vi "Stimulus Channel (G3)-Serialize.vi"(8 "error in":errorcluster, 11 "variant":variant) -> (0 "error out":errorcluster, 1 "Cluster Data Types":variant[](array[variant]), 3 "Cluster Variants":variant[](array[variant]))   [LabVIEW 2020, in "Stimulus Channel (G3).xctl"]
uses:
  Stimulus Channel (G3).xctl
  Waveform VIs/Complex Tone VIs/CT.Properties.ctl
  Waveform VIs/Complex Tone VIs/CT-Phase Enum.ctl
  Level (G3)/Level.Properties.ctl
  Level (G3)/Level Units (G3).ctl
  Full Stimulus Channel Data.ctl
  Waveform XControls/Waveform (G3)/Waveform Data.ctl
  Waveform VIs/Waveform Enum (V3).ctl
  Waveform XControls/Tone (G3)/Tone.Properties.ctl
  Waveform VIs/Pulse Train VIs/Pulse Train Params.ctl
  Waveform VIs/Pulse Train VIs/Pulse Polarity.ctl
  Waveform VIs/Pulse Train VIs/PT-Continuous State.ctl
  Waveform VIs/Noise VIs/Noise (G3).ctl
  Waveform VIs/Noise VIs/Noise (G3).Properties.ctl
  Waveform VIs/Noise VIs/Noise (G3).Data.ctl
  Waveform VIs/File VIs/StimFile-Params.ctl
  Waveform VIs/FM Sweep VIs/FM Sweep Params.ctl
  Waveform VIs/Chirp Train VIs/Chirp Train.ctl
  Waveform VIs/Chirp Train VIs/Chirp Train Params.ctl
  Waveform VIs/Complex Tone VIs/CT-Params.ctl
  Waveform VIs/Complex Tone VIs/CT-Runtime Data.ctl
  Waveform XControls/FM Tone/Data.ctl
  Waveform XControls/Vowel/Vowel.Properties.ctl
  Waveform VIs/Ramp VIs/Ramp.Properties.ctl
  Filter (G3)/Filter Data.ctl
  Filter (G3)/Filter Type.ctl
  Filter VIs/Filter-Bandwidth Units.ctl
  Controls/Burst XCtl/Burst Data.ctl
  Level (G3)/Level Data.ctl
  Advanced Options (G3)/Advanced Options (G3).ctl
  Modulation VIs/SAM VIs/SAM Params.ctl
  Typedefs/Destination.ctl
  Modulation VIs/SAM VIs/SAM.Properties.ctl
  Controls/Waveform XCtl/Waveform Enum.ctl
  Waveform VIs/Tone VIs/Tone.Properties.ctl
  Waveform VIs/Pulse Train VIs/Pulse Train.Properties.ctl
  Waveform VIs/File VIs/File.Properties.ctl
  Waveform VIs/FM Sweep VIs/FMSweep.Properties.ctl
  Waveform VIs/Chirp Train VIs/Chirp Train.Properties.ctl
  Waveform XControls/FM Tone/FM.Properties.ctl
  Waveform XControls/Waveform (G3)/Waveform (G3).xctl
  Filter (G3)/Filter (G3).xctl
  Controls/Burst XCtl/Burst Control.xctl
  Level (G3)/Level (G3).xctl
  <vilib>/Utility/Data Type/NI_Data Type.lvlib
  Advanced Options (G3)/Advanced Options (G3).xctl
  Waveform XControls/Tone (G3)/Tone (G3).xctl
  Waveform XControls/FM Tone/FM Tone.xctl
  Waveform XControls/Vowel/Vowel.xctl
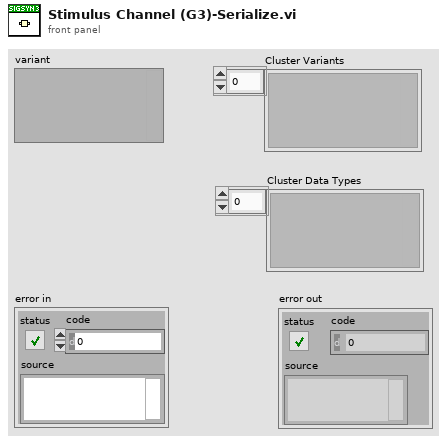
[diagram p1: front panel]
types:
  T1 = typedef "CT.Properties.ctl" = cluster{"F0 (Hz)":dbl, "Band":cluster{"Flow (Hz)":dbl, "Fhigh (Hz)":dbl}, "Phase":T2, "Min F0 (Hz)":dbl, "Max F0 (Hz)":dbl, "ContinRandPhase":bool, "Max peak factor":dbl, "Max mod depth":dbl, "MinHarmNum":i32, "MaxHarmNum":i32, "Level Mode":enum16{"per component", "overall rms"}}
  T2 = typedef "CT-Phase Enum.ctl" = enum16{"Cosine", "Random", "Alternating"}
  T3 = typedef "Level.Properties.ctl" = cluster{"Level":dbl, "Units":T4}
  T4 = typedef "Level (G3).xctl/Level Units (G3).ctl" = enum16{"dB atten", "dB SPL", "dB re 1 Vrms", "dB V/Hz½", "mW", "dB HL", "Volts", "dB mW"}
  T5 = typedef "Stimulus Channel (G3).xctl/Full Stimulus Channel Data.ctl" = cluster{"Waveform":T6, "Filter":T24, "Burst":T27, "Level":T28, "Name":string, "Advanced":T29, "SAM":T30, "Destination":T31}
  T6 = typedef "Waveform (G3).xctl/Waveform Data.ctl" = cluster{"Type":T7, "Tone":T8, "Pulse Train":T9, "Noise":T12, "File":T15, "FMSweep":T16, "Chirp Train":T17, "Complex Tone":cluster{"Params":T19, "Data":T20}, "FM":T21, "Vowel":T22, "Ramp":T23}
  T7 = typedef "Waveform Enum (V3).ctl" = enum16{"OFF", "Tone", "Noise", "Pulse Train", "File", "FM Sweep", "Chirp Train", "Complex Tone", "FM Tone", "Vowel", "Ramp"}
  T8 = typedef "Tone (G3).xctl/Tone.Properties.ctl" = cluster{"Frequency (kHz)":dbl, "Phase (cycles)":dbl, "Random phase":bool}
  T9 = typedef "Pulse Train Params.ctl" = cluster{"Pulse width (us)":dbl, "Pulse rate (Hz)":dbl, "Gap (ms)":dbl, "Polarity":T10, "PT State":T11, "Asynch":bool}
  T10 = typedef "Pulse Polarity.ctl" = enum16{"POS", "NEG", "POS-NEG", "NEG-POS"}
  T11 = typedef "PT-Continuous State.ctl" = cluster{"Template":dbl[], "Nperiod":i32, "Index":i32, "Pulse Rate (Hz)":dbl, "Phase (cycles)":dbl, "Noff":i32}
  T12 = typedef "Noise (G3).ctl" = cluster{"Properties":T13, "Data":T14}
  T13 = typedef "Noise (G3).Properties.ctl" = cluster{"InvFilt":bool, "Aweight":bool, "Seed":i32, "Tokens":i32, "Brickwall":bool}
  T14 = typedef "Noise (G3).Data.ctl" = cluster{"TokenNum":i32}
  T15 = typedef "StimFile-Params.ctl" = cluster{"Filename":path, "Signal":dbl[], "Channel":i32, "stream":bool, "offset":i32, "nreps":i32, "loops":i32, "Randomize":bool, "order":i32[], "Seed":i32, "Tokens":i32}
  T16 = typedef "FM Sweep Params.ctl" = cluster{"Rate (oct/s)":dbl, "Fmin (Hz)":dbl, "Fmax (Hz)":dbl, "Ramp (ms)":dbl, "Linear":bool}
  T17 = typedef "Chirp Train.ctl" = cluster{"Params":T18, "Data":cluster{"WF":dbl[]}}
  T18 = typedef "Chirp Train Params.ctl" = cluster{"Fmin (kHz)":dbl, "Fmax (kHz)":dbl, "Compensate":bool, "Duration (ms)":dbl}
  T19 = typedef "CT-Params.ctl" = cluster{"F0 (Hz)":dbl, "Band":cluster{"Flow (Hz)":dbl, "Fhigh (Hz)":dbl}, "Phase":T2, "Min F0 (Hz)":dbl, "Max F0 (Hz)":dbl, "ContinRandPhase":bool, "Max peak factor":dbl, "Max mod depth":dbl, "MinHarmNum":i32, "MaxHarmNum":i32, "Level Mode":enum16{"per component", "overall rms"}, "% jitter":dbl}
  T20 = typedef "CT-Runtime Data.ctl" = cluster{"Ncomp":i32, "MinHarm":i32, "Phase":dbl[], "Amplitude":dbl[], "Npts/frame":i32, "Last F0":dbl, "Fmin":dbl, "Fmax":dbl, "Lslope":dbl, "randphase":bool, "overall rms":bool, "fmult":dbl[], "jittered":bool}
  T21 = typedef "FM Tone.xctl/Data.ctl" = cluster{"Carrier (kHz)":dbl, "ModRate (Hz)":dbl, "Depth (Hz)":dbl, "Phase (cycles)":dbl}
  T22 = typedef "Vowel.xctl/Vowel.Properties.ctl" = cluster{"Freqs":string, "Set level":enum16{"Total", "Per component"}, "Freq":dbl[], "weights":dbl[]}
  T23 = typedef "Ramp.Properties.ctl" = cluster{"Duration (ms)":dbl}
  T24 = typedef "Filter (G3).xctl/Filter Data.ctl" = cluster{"Type":T25, "CF (kHz)":dbl, "BW (kHz)":dbl, "Cascade":bool, "Quadrature":bool, "Scale Factor":dbl, "Stages":cluster{"IIR Filter":cluster{"filter structure":enum32{"IIR 2nd Order", "IIR 4th Order"}, "Reverse Coefficients":dbl[], "Forward Coefficients":dbl[]}, "State":dbl[]}[], "Class":enum16{"Elliptic", "Butterworth"}, "Order":i32, "BWUnits":T26}
  T25 = typedef "Filter (G3).xctl/Filter Type.ctl" = enum16{"OFF", "Lowpass", "Highpass", "Bandpass", "Bandstop"}
  T26 = typedef "Filter-Bandwidth Units.ctl" = enum16{"Linear", "Octaves", "Min-Max"}
  T27 = typedef "Burst Control.xctl/Burst Data.ctl" = cluster{"Active":bool, "Delay (ms)":dbl, "Duration (ms)":dbl, "Ramp (ms)":dbl, "Rate (Hz)":dbl, "Trepeat (ms)":dbl, "Repeat":bool}
  T28 = typedef "Level (G3).xctl/Level Data.ctl" = cluster{"Level":dbl, "Units":T4, "Max":dbl, "Data":cluster{"Multiplier":dbl, "Cal File":path, "Cal":cluster{"Freq (Hz)":dbl[], "Mag (dB SPL)":dbl[], "Phase (deg)":dbl[]}, "audiogram":path}}
  T29 = typedef "Advanced Options (G3).xctl/Advanced Options (G3).ctl" = cluster{"AltPol":bool, "Var":string, "Expr":string}
  T30 = typedef "SAM Params.ctl" = cluster{"Active":bool, "Frequency (Hz)":dbl, "Depth":dbl, "Init Phase (cycles)":dbl, "phase (degrees)":dbl, "Asynch":bool}
  T31 = typedef "Destination.ctl" = cluster{"Name":string, "Num":i32}
  T32 = typedef "Waveform Enum.ctl" = enum16{"OFF", "Tone", "Noise", "Pulse Train", "File", "FM Sweep", "Chirp Train", "Complex Tone", "FM Tone", "Moving Ripple"}
  T33 = typedef "Tone.Properties.ctl" = cluster{"Frequency (kHz)":dbl, "Phase (cycles)":dbl, "Random phase":bool}
  T34 = typedef "Pulse Train.Properties.ctl" = cluster{"Pulse width (us)":dbl, "Pulse rate (Hz)":dbl, "Gap (ms)":dbl, "Polarity":T10, "Asynch":bool}
  T35 = typedef "File.Properties.ctl" = cluster{"Filename":path, "Channel":i32, "Tokens":i32, "Randomize":bool, "Seed":i32}
  T36 = typedef "FMSweep.Properties.ctl" = cluster{"Rate (oct/s)":dbl, "Fmin (Hz)":dbl, "Fmax (Hz)":dbl, "Ramp (ms)":dbl, "Linear":bool}
  T37 = typedef "Chirp Train.Properties.ctl" = cluster{"Fmin (kHz)":dbl, "Fmax (kHz)":dbl, "Compensate":bool, "Duration (ms)":dbl}
  T38 = typedef "FM Tone.xctl/FM.Properties.ctl" = cluster{"Carrier (kHz)":dbl, "ModRate (Hz)":dbl, "Depth (Hz)":dbl, "Phase (cycles)":dbl}
  T39 = cluster{"Active":bool, "Delay (ms)":dbl, "Duration (ms)":dbl, "Ramp (ms)":dbl, "Repeat":bool}
  T40 = typedef "SAM.Properties.ctl" = cluster{"Active":bool, "Frequency (Hz)":dbl, "Depth":dbl, "Init Phase (cycles)":dbl, "Asynch":bool}
  T41 = typedef "NI_Data Type.lvlib/Data Type.ctl" = enum8{"Invalid Type", "Void", "I8", "I16", "I32", "I64", "U8", "U16", "U32", "U64", "Single Float", "Double Float", "Extended Float", "Single Complex", "Double Complex", "Extended Complex", "Enum U8", "Enum U16", "Enum U32", "Enum U64", "Single Float With Unit", "Double Float With Unit", "Extended Float With Unit", "Single Complex with Unit", "Double Complex with Unit", "Extended Complex with Unit", "Boolean", "String", "Path", "Picture", "Tag", "Array", "Cluster", "Variant", "LV Variant", "Waveform", "Timestamp", "Digital Waveform", "Digital Data", "ExpressData", "Refnum", "External Data", "VI", "Poly VI", "LabVIEW Class Instance", "Fixed Point", "Set Collection", "Map Collection"}
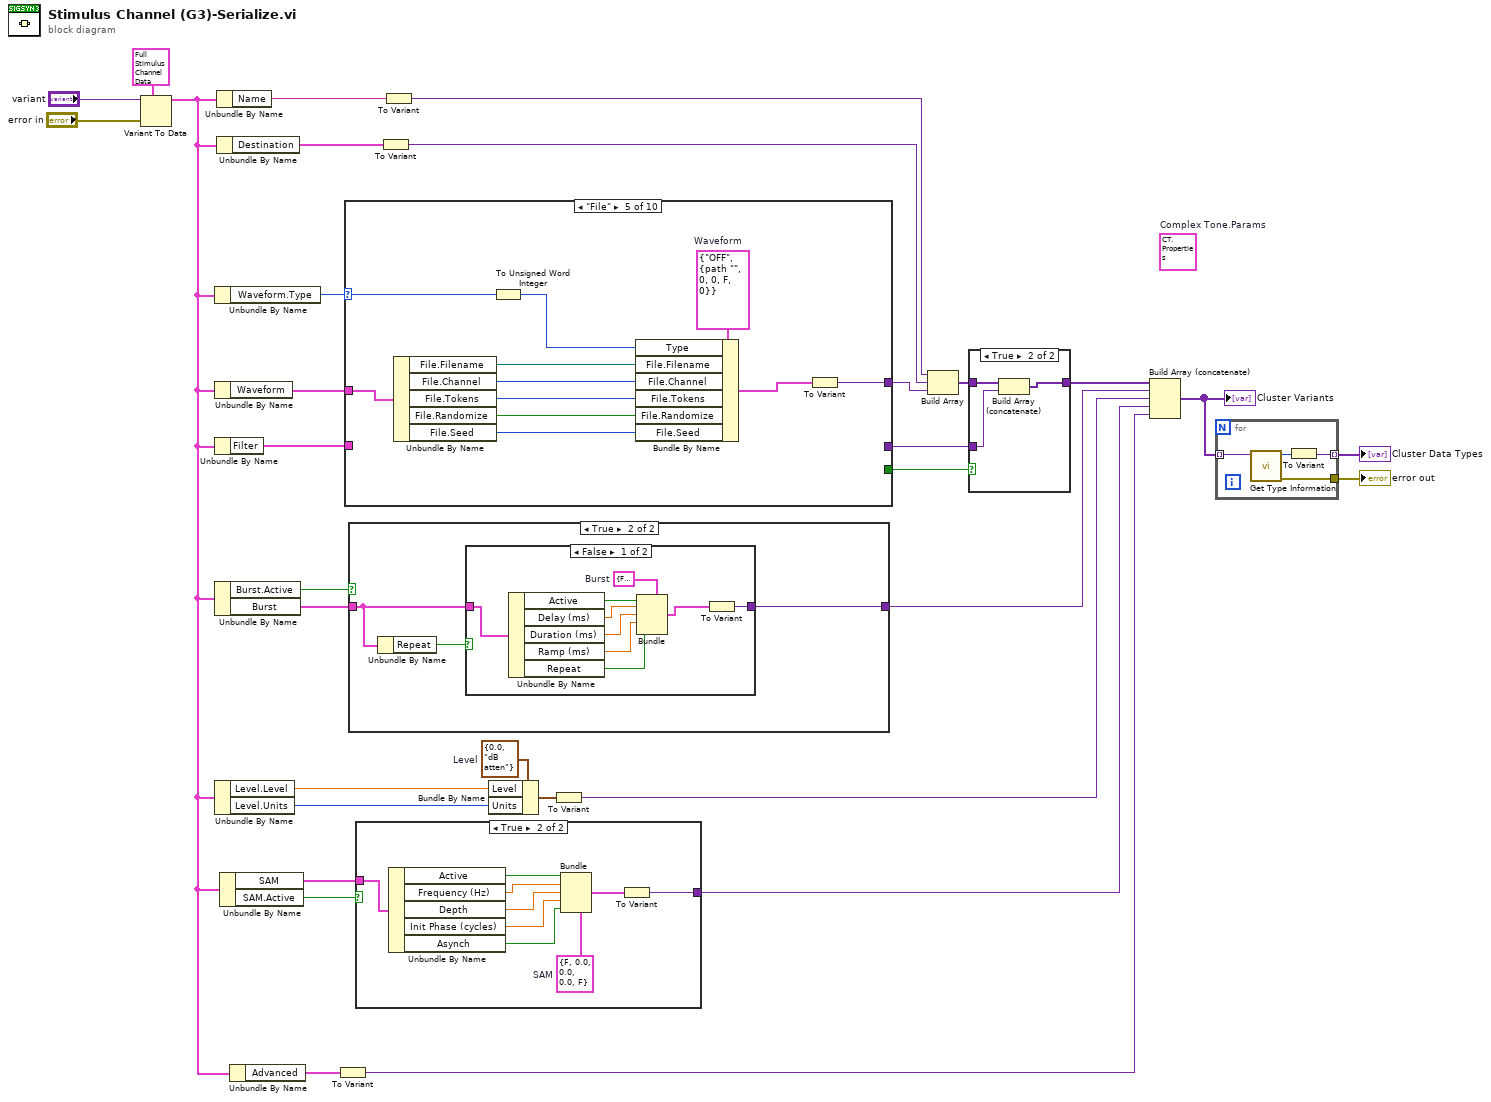
[diagram p0: block diagram]
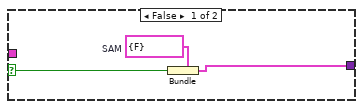
[diagram p2: hidden frame]
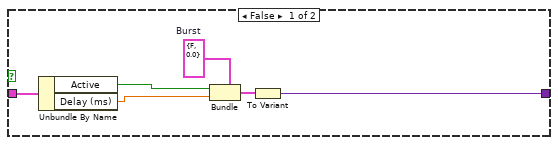
[diagram p3: hidden frame]
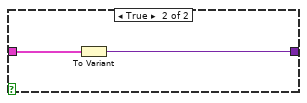
[diagram p4: hidden frame]
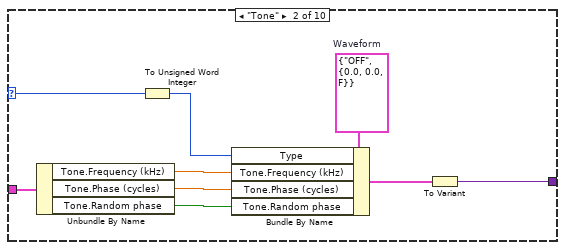
[diagram p7: hidden frame]
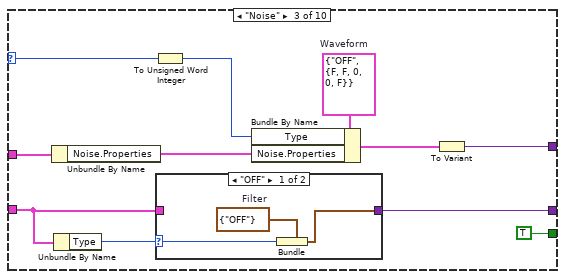
[diagram p8: hidden frame]
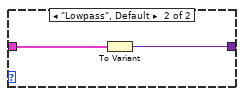
[diagram p9: hidden frame]
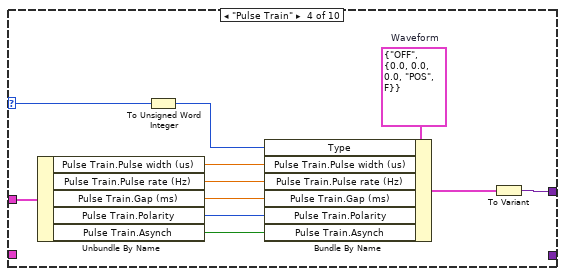
[diagram p10: hidden frame]
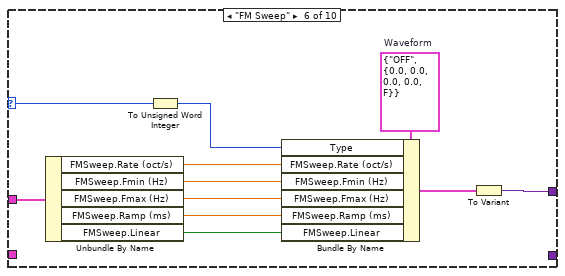
[diagram p11: hidden frame]
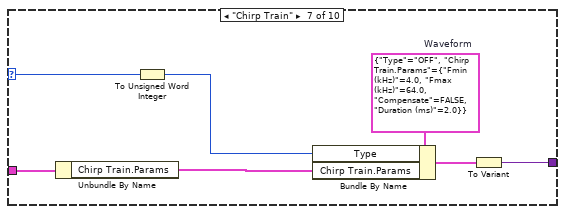
[diagram p12: hidden frame]
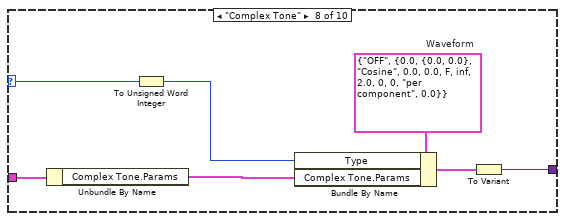
[diagram p13: hidden frame]
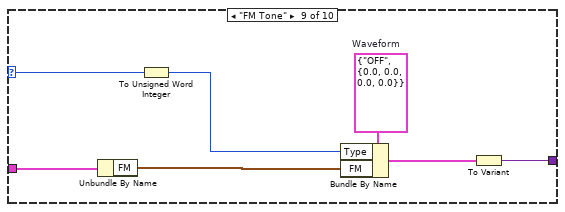
[diagram p14: hidden frame]
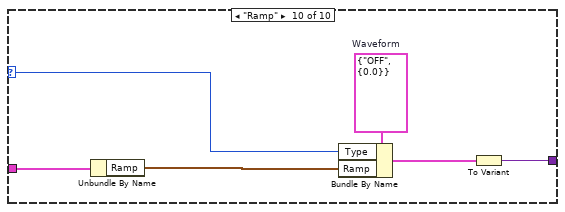
[diagram p15: hidden frame]
diagram:
  (unwired) T1 {"F0 (Hz)"=0.0, "Band"={"Flow (Hz)"=0.0, "Fhigh (Hz)"=0.0}, "Phase"=enum."Cosine", "Min F0 (Hz)"=0.0, "Max F0 (Hz)"=0.0, "ContinRandPhase"=FALSE, "Max peak factor"=inf, "Max mod depth"=2.0, "MinHarmNum"=0, "MaxHarmNum"=0, "Level Mode"=enum."per component"}  # Complex Tone.Params
  w11 = T3 {"Level"=0.0, "Units"=enum."dB atten"}  # Level
  n1 = Variant To Data(error in="error in", type=T5 {"Waveform"={"Type"=enum."Tone", "Tone"={"Frequency (kHz)"=0.0, "Phase (cycles)"=0.0, "Random phase"=FALSE}, "Pulse Train"={"Pulse width (us)"=0.0, "Pulse rate (Hz)"=0.0, "Gap (ms)"=0.0, "Polarity"=enum."POS", "PT State"={"Template"=[], "Nperiod"=0, "Index"=0, "Pulse Rate (Hz)"=0.0, "Phase (cycles)"=0.0, "Noff"=0}, "Asynch"=FALSE}, "Noise"={"Properties"={"InvFilt"=FALSE, "Aweight"=FALSE, "Seed"=0, "Tokens"=0, "Brickwall"=FALSE}, "Data"={"TokenNum"=0}}, "File"={"Filename"=path "", "Signal"=[], "Channel"=0, "stream"=FALSE, "offset"=0, "nreps"=0, "loops"=0, "Randomize"=FALSE, "order"=[], "Seed"=0, "Tokens"=0}, "FMSweep"={"Rate (oct/s)"=0.0, "Fmin (Hz)"=0.0, "Fmax (Hz)"=0.0, "Ramp (ms)"=0.0, "Linear"=FALSE}, "Chirp Train"={"Params"={"Fmin (kHz)"=4.0, "Fmax (kHz)"=64.0, "Compensate"=FALSE, "Duration (ms)"=2.0}, "Data"={"WF"=[]}}, "Complex Tone"={"Params"={"F0 (Hz)"=0.0, "Band"={"Flow (Hz)"=0.0, "Fhigh (Hz)"=0.0}, "Phase"=enum."Cosine", "Min F0 (Hz)"=0.0, "Max F0 (Hz)"=0.0, "ContinRandPhase"=FALSE, "Max peak factor"=inf, "Max mod depth"=2.0, "MinHarmNum"=0, "MaxHarmNum"=0, "Level Mode"=enum."per component", "% jitter"=0.0}, "Data"={"Ncomp"=0, "MinHarm"=0, "Phase"=[], "Amplitude"=[], "Npts/frame"=0, "Last F0"=0.0, "Fmin"=0.0, "Fmax"=0.0, "Lslope"=0.0, "randphase"=FALSE, "overall rms"=FALSE, "fmult"=[], "jittered"=FALSE}}, "FM"={"Carrier (kHz)"=0.0, "ModRate (Hz)"=0.0, "Depth (Hz)"=0.0, "Phase (cycles)"=0.0}, "Vowel"={"Freqs"="", "Set level"=enum."Total", "Freq"=[], "weights"=[]}, "Ramp"={"Duration (ms)"=0.0}}, "Filter"={"Type"=enum."Lowpass", "CF (kHz)"=0.0, "BW (kHz)"=0.0, "Cascade"=FALSE, "Quadrature"=FALSE, "Scale Factor"=0.0, "Stages"=[], "Class"=enum."Elliptic", "Order"=0, "BWUnits"=enum."Linear"}, "Burst"={"Active"=FALSE, "Delay (ms)"=0.0, "Duration (ms)"=0.0, "Ramp (ms)"=0.0, "Rate (Hz)"=0.0, "Trepeat (ms)"=0.0, "Repeat"=FALSE}, "Level"={"Level"=0.0, "Units"=enum."dB atten", "Max"=0.0, "Data"={"Multiplier"=0.0, "Cal File"=path "", "Cal"={"Freq (Hz)"=[], "Mag (dB SPL)"=[], "Phase (deg)"=[]}, "audiogram"=path ""}}, "Name"="", "Advanced"={"AltPol"=FALSE, "Var"="", "Expr"=""}, "SAM"={"Active"=FALSE, "Frequency (Hz)"=0.0, "Depth"=0.0, "Init Phase (cycles)"=0.0, "phase (degrees)"=0.0, "Asynch"=FALSE}, "Destination"={"Name"="", "Num"=0}} ("StimChan"), Variant="variant") -> (data=w3:T5)  [unwired: 1 out]
  n2 = Unbundle By Name(w3) -> ("Waveform.Type"=w30:T7)
  n3 = Unbundle By Name(w3) -> ("Waveform"=w29:T6)
  n4 = Unbundle By Name(w3) -> ("Filter"=w20:T24)
  n5 = Unbundle By Name(w3) -> ("Burst.Active"=w14:bool, "Burst"=w13:T27)
  n6 = Unbundle By Name(w3) -> ("Level.Level"=w10:dbl, "Level.Units"=w9:T4)
  n7 = Unbundle By Name(w3) -> ("Name"=w25:string)
  n8 = Unbundle By Name(w3) -> ("Destination"=w23:T31)
  n9 = Unbundle By Name(w3) -> ("SAM"=w5:T30, "SAM.Active"=w6:bool)
  n10 = Unbundle By Name(w3) -> ("Advanced"=w2:T29)
  n11 = To Variant(anything=w2) -> (Variant=w1:variant)
  n12 = case shown="\"File\"" w30 {
    selector: w30 -> [_ w40 w51 w67 w78 w89 w96 w103 w110 w116]
    tunnel: w29 -> [_ w41 w52 w68 w79 w90 w97 w104 w111 w117]
    tunnel: [_ w38 w47 w65 w76 w87 w94 w101 w108 w114] -> w28
    tunnel: [_ _ w45 _ _ _ _ _ _ _] -> w18
    tunnel: w20 -> [_ _ w44 _ _ _ _ _ _ _]
    tunnel: [_ _ TRUE _ _ _ _ _ _ _] -> w19
    frame "OFF", Default {
    }
    frame "Tone" {
      w37 = cluster{"Type":T32, "Tone":T33} {"Type"=enum."OFF", "Tone"={"Frequency (kHz)"=0.0, "Phase (cycles)"=0.0, "Random phase"=FALSE}}  # Waveform
      n13 = Unbundle By Name(w41) -> ("Tone.Frequency (kHz)"=w36:dbl, "Tone.Phase (cycles)"=w35:dbl, "Tone.Random phase"=w34:bool)
      n14 = To Unsigned Word Integer(number=w40) -> (unsigned 16bit integer=w33:u16)
      n15 = Bundle By Name(cluster=w37, "Type"=w33, "Tone.Frequency (kHz)"=w36, "Tone.Phase (cycles)"=w35, "Tone.Random phase"=w34) -> (w39:cluster{"Type":T32, "Tone":T33})
      n16 = To Variant(anything=w39) -> (Variant=w38:variant)
    }
    frame "Noise" {
      w49 = cluster{"Type":T32, "Noise.Properties":T13} {"Type"=enum."OFF", "Noise.Properties"={"InvFilt"=FALSE, "Aweight"=FALSE, "Seed"=0, "Tokens"=0, "Brickwall"=FALSE}}  # Waveform
      n17 = Unbundle By Name(w52) -> ("Noise.Properties"=w48:T13)
      n18 = Unbundle By Name(w44) -> ("Type"=w46:T25)
      n19 = To Unsigned Word Integer(number=w51) -> (unsigned 16bit integer=w42:u16)
      n20 = case shown="\"OFF\"" w46 {
        selector: w46 -> [w55 _]
        tunnel: w44 -> [_ w57]
        tunnel: [w53 w56] -> w45
        frame "OFF" {
          w54 = cluster{"Type":T25} {"Type"=enum."OFF"}  # Filter
          n21 = Bundle(cluster=w54, "Type"=w55) -> (w53:cluster{"Type":T25})
        }
        frame "Lowpass", Default {
          n22 = To Variant(anything=w57) -> (Variant=w56:variant)
        }
      }
      n23 = Bundle By Name(cluster=w49, "Type"=w42, "Noise.Properties"=w48) -> (w50:cluster{"Type":T32, "Noise.Properties":T13})
      n24 = To Variant(anything=w50) -> (Variant=w47:variant)
    }
    frame "Pulse Train" {
      w64 = cluster{"Type":T32, "Pulse Train":T34} {"Type"=enum."OFF", "Pulse Train"={"Pulse width (us)"=0.0, "Pulse rate (Hz)"=0.0, "Gap (ms)"=0.0, "Polarity"=enum."POS", "Asynch"=FALSE}}  # Waveform
      n25 = Unbundle By Name(w68) -> ("Pulse Train.Pulse width (us)"=w63:dbl, "Pulse Train.Pulse rate (Hz)"=w62:dbl, "Pulse Train.Gap (ms)"=w61:dbl, "Pulse Train.Polarity"=w60:T10, "Pulse Train.Asynch"=w59:bool)
      n26 = To Unsigned Word Integer(number=w67) -> (unsigned 16bit integer=w58:u16)
      n27 = Bundle By Name(cluster=w64, "Type"=w58, "Pulse Train.Pulse width (us)"=w63, "Pulse Train.Pulse rate (Hz)"=w62, "Pulse Train.Gap (ms)"=w61, "Pulse Train.Polarity"=w60, "Pulse Train.Asynch"=w59) -> (w66:cluster{"Type":T32, "Pulse Train":T34})
      n28 = To Variant(anything=w66) -> (Variant=w65:variant)
    }
    frame "File" {
      w75 = cluster{"Type":T32, "File":T35} {"Type"=enum."OFF", "File"={"Filename"=path "", "Channel"=0, "Tokens"=0, "Randomize"=FALSE, "Seed"=0}}  # Waveform
      n29 = Unbundle By Name(w79) -> ("File.Filename"=w74:path, "File.Channel"=w73:i32, "File.Tokens"=w71:i32, "File.Randomize"=w70:bool, "File.Seed"=w69:i32)
      n30 = To Unsigned Word Integer(number=w78) -> (unsigned 16bit integer=w72:u16)
      n31 = Bundle By Name(cluster=w75, "Type"=w72, "File.Filename"=w74, "File.Channel"=w73, "File.Tokens"=w71, "File.Randomize"=w70, "File.Seed"=w69) -> (w77:cluster{"Type":T32, "File":T35})
      n32 = To Variant(anything=w77) -> (Variant=w76:variant)
    }
    frame "FM Sweep" {
      w86 = cluster{"Type":T32, "FMSweep":T36} {"Type"=enum."OFF", "FMSweep"={"Rate (oct/s)"=0.0, "Fmin (Hz)"=0.0, "Fmax (Hz)"=0.0, "Ramp (ms)"=0.0, "Linear"=FALSE}}  # Waveform
      n33 = Unbundle By Name(w90) -> ("FMSweep.Rate (oct/s)"=w85:dbl, "FMSweep.Fmin (Hz)"=w81:dbl, "FMSweep.Fmax (Hz)"=w82:dbl, "FMSweep.Ramp (ms)"=w83:dbl, "FMSweep.Linear"=w84:bool)
      n34 = To Unsigned Word Integer(number=w89) -> (unsigned 16bit integer=w80:u16)
      n35 = Bundle By Name(cluster=w86, "Type"=w80, "FMSweep.Rate (oct/s)"=w85, "FMSweep.Fmin (Hz)"=w81, "FMSweep.Fmax (Hz)"=w82, "FMSweep.Ramp (ms)"=w83, "FMSweep.Linear"=w84) -> (w88:cluster{"Type":T32, "FMSweep":T36})
      n36 = To Variant(anything=w88) -> (Variant=w87:variant)
    }
    frame "Chirp Train" {
      w93 = cluster{"Type":T32, "Chirp Train.Params":T37} {"Type"=enum."OFF", "Chirp Train.Params"={"Fmin (kHz)"=4.0, "Fmax (kHz)"=64.0, "Compensate"=FALSE, "Duration (ms)"=2.0}}  # Waveform
      n37 = Unbundle By Name(w97) -> ("Chirp Train.Params"=w92:T18)
      n38 = To Unsigned Word Integer(number=w96) -> (unsigned 16bit integer=w91:u16)
      n39 = Bundle By Name(cluster=w93, "Type"=w91, "Chirp Train.Params"=w92) -> (w95:cluster{"Type":T32, "Chirp Train.Params":T37})
      n40 = To Variant(anything=w95) -> (Variant=w94:variant)
    }
    frame "Complex Tone" {
      w100 = cluster{"Type":T32, "Complex Tone.Params":T19} {"Type"=enum."OFF", "Complex Tone.Params"={"F0 (Hz)"=0.0, "Band"={"Flow (Hz)"=0.0, "Fhigh (Hz)"=0.0}, "Phase"=enum."Cosine", "Min F0 (Hz)"=0.0, "Max F0 (Hz)"=0.0, "ContinRandPhase"=FALSE, "Max peak factor"=inf, "Max mod depth"=2.0, "MinHarmNum"=0, "MaxHarmNum"=0, "Level Mode"=enum."per component", "% jitter"=0.0}}  # Waveform
      n41 = Unbundle By Name(w104) -> ("Complex Tone.Params"=w99:T19)
      n42 = To Unsigned Word Integer(number=w103) -> (unsigned 16bit integer=w98:u16)
      n43 = Bundle By Name(cluster=w100, "Type"=w98, "Complex Tone.Params"=w99) -> (w102:cluster{"Type":T32, "Complex Tone.Params":T19})
      n44 = To Variant(anything=w102) -> (Variant=w101:variant)
    }
    frame "FM Tone" {
      w107 = cluster{"Type":T32, "FM":T38} {"Type"=enum."OFF", "FM"={"Carrier (kHz)"=0.0, "ModRate (Hz)"=0.0, "Depth (Hz)"=0.0, "Phase (cycles)"=0.0}}  # Waveform
      n45 = Unbundle By Name(w111) -> ("FM"=w106:T21)
      n46 = To Unsigned Word Integer(number=w110) -> (unsigned 16bit integer=w105:u16)
      n47 = Bundle By Name(cluster=w107, "Type"=w105, "FM"=w106) -> (w109:cluster{"Type":T32, "FM":T38})
      n48 = To Variant(anything=w109) -> (Variant=w108:variant)
    }
    frame "Ramp" {
      w113 = cluster{"Type":T7, "Ramp":T23} {"Type"=enum."OFF", "Ramp"={"Duration (ms)"=0.0}}  # Waveform
      n49 = Unbundle By Name(w117) -> ("Ramp"=w112:T23)
      n50 = Bundle By Name(cluster=w113, "Type"=w116, "Ramp"=w112) -> (w115:cluster{"Type":T7, "Ramp":T23})
      n51 = To Variant(anything=w115) -> (Variant=w114:variant)
    }
  }
  n52 = case shown="True" w14 {
    tunnel: w13 -> [w123 w125]
    tunnel: [w118 w124] -> w12
    frame False {
      w120 = cluster{"Active":bool, "Delay (ms)":dbl} {"Active"=FALSE, "Delay (ms)"=0.0}  # Burst
      n53 = Unbundle By Name(w123) -> ("Active"=w122:bool, "Delay (ms)"=w121:dbl)
      n54 = Bundle(cluster=w120, "Active"=w122, "Delay (ms)"=w121) -> (w119:cluster{"Active":bool, "Delay (ms)":dbl})
      n55 = To Variant(anything=w119) -> (Variant=w118:variant)
    }
    frame True {
      n56 = Unbundle By Name(w125) -> ("Repeat"=w126:bool)
      n57 = case shown="False" w126 {
        tunnel: w125 -> [w135 w137]
        tunnel: [w128 w136] -> w124
        frame False {
          w127 = T39 {"Active"=FALSE, "Delay (ms)"=0.0, "Duration (ms)"=0.0, "Ramp (ms)"=0.0, "Repeat"=FALSE}  # Burst
          n58 = Unbundle By Name(w135) -> ("Active"=w134:bool, "Delay (ms)"=w133:dbl, "Duration (ms)"=w132:dbl, "Ramp (ms)"=w131:dbl, "Repeat"=w130:bool)
          n59 = Bundle(cluster=w127, "Active"=w134, "Delay (ms)"=w133, "Duration (ms)"=w132, "Ramp (ms)"=w131, "Repeat"=w130) -> (w129:T39)
          n60 = To Variant(anything=w129) -> (Variant=w128:variant)
        }
        frame True {
          n61 = To Variant(anything=w137) -> (Variant=w136:variant)
        }
      }
    }
  }
  n62 = case shown="True" w6 {
    selector: w6 -> [w140 _]
    tunnel: w5 -> [_ w149]
    tunnel: [w138 w141] -> w4
    frame False {
      w139 = cluster{"Active":bool} {"Active"=FALSE}  # SAM
      n63 = Bundle(cluster=w139, "Active"=w140) -> (w138:cluster{"Active":bool})
    }
    frame True {
      w143 = T40 {"Active"=FALSE, "Frequency (Hz)"=0.0, "Depth"=0.0, "Init Phase (cycles)"=0.0, "Asynch"=FALSE}  # SAM
      n64 = Unbundle By Name(w149) -> ("Active"=w148:bool, "Frequency (Hz)"=w147:dbl, "Depth"=w146:dbl, "Init Phase (cycles)"=w145:dbl, "Asynch"=w144:bool)
      n65 = Bundle(cluster=w143, "Active"=w148, "Frequency (Hz)"=w147, "Depth"=w146, "Init Phase (cycles)"=w145, "Asynch"=w144) -> (w142:T40)
      n66 = To Variant(anything=w142) -> (Variant=w141:variant)
    }
  }
  n67 = To Variant(anything=w23) -> (Variant=w22:variant)
  n68 = To Variant(anything=w25) -> (Variant=w24:variant)
  n69 = Bundle By Name(cluster=w11, "Level"=w10, "Units"=w9) -> (w8:T3)
  n70 = To Variant(anything=w8) -> (Variant=w7:variant)
  n71 = Build Array(w24, w22, w28) -> (w17:variant[])
  n72 = case shown="True" w19 {
    tunnel: w18 -> [_ w152]
    tunnel: w17 -> [w150 w153]
    tunnel: [w150 w151] -> w16
    frame False {
    }
    frame True {
      n73 = Build Array (concatenate)(w153, w152) -> (w151:variant[])
    }
  }
  n74 = Build Array (concatenate)(w16, w12, w7, w4, w1) -> (w15:variant[])
  "Cluster Variants" <- w15
  n75 = for {
    tunnel: [w156] -> w26
    tunnel: w15 -> [w155] mode=indexing
    tunnel: [w154] -> w21 mode=indexing
    n76 = call <vilib>:"Get Type Information.vi"("variant"=w155) -> ("error out"=w156:errorcluster, "type"=w157:T41)  [unwired: 6 in, 3 out]
    n77 = To Variant(anything=w157) -> (Variant=w154:variant)
  }
  "Cluster Data Types" <- w21
  "error out" <- w26
